vi "Unmarshal.vi"(8 "error in (no error)":errorcluster, 10 "Buffer":u8[](array[numeric]), 11 "LEN in":refnum<class "LEN.lvclass">) -> (0 "error out":errorcluster, 2 "Buffer Count":i32, 3 "LEN out":refnum<class "LEN.lvclass">)   [LabVIEW 2020, in "Protobuf RAW.lvlib" / "LEN.lvclass"]
uses:
  LEN.lvclass
  bytes/bytes.lvclass
  E:/Labview/LV 2020/Libs/LV Protobuf Raw/Source/Proto Encode/LEN Encoder/LEN.lvclass
  Message/Raw Message.lvclass
  string/string.lvclass
  E:/Labview/LV 2020/Libs/LV Protobuf Raw/Source/Proto Type Common/Proto Type Common.lvclass
  E:/Labview/LV 2020/Libs/LV Protobuf Raw/Source/Protobuf RAW/Tag/Basic Type.lvclass
  E:/Labview/LV 2020/Libs/LV Protobuf Raw/Source/Protobuf RAW/Proto Value/Proto Type.lvclass
  E:/Labview/LV 2020/Libs/LV Protobuf Raw/Source/Protobuf RAW/Type Serializer/Type Serializer.lvclass
  E:/Labview/LV 2020/Libs/LV Protobuf Raw/Source/Protobuf RAW/String Representable/String Representable.lvclass
  E:/Labview/LV 2020/Libs/LV Protobuf Raw/Source/Protobuf RAW/Wire Type Group/Wire Type Group.lvclass
  E:/Labview/LV 2020/Libs/LV Protobuf Raw/Source/Protobuf RAW/LEN Encoder/LEN.lvclass
  E:/Labview/LV 2020/Libs/LV Protobuf Raw/Source/Protobuf RAW/string/string.lvclass
  E:/Labview/LV 2020/Libs/LV Protobuf Raw/Source/Protobuf RAW/Message/Raw Message.lvclass
  E:/Labview/LV 2020/Libs/LV Protobuf Raw/Source/Protobuf RAW/bytes/bytes.lvclass
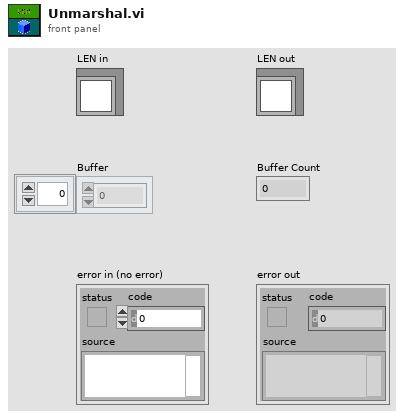
[diagram p1: front panel]
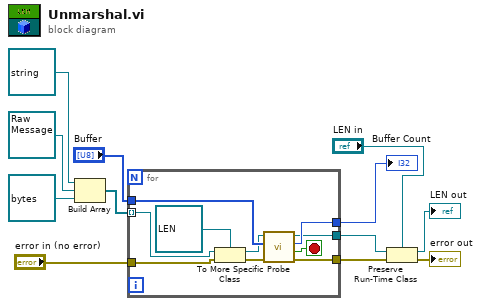
[diagram p0: block diagram]
diagram:
  n1 = Build Array(refnum<class "string.lvclass"> refnum ("Protobuf Encode.lvlib:string.lvclass"), refnum<class "Raw Message.lvclass"> refnum ("Protobuf Encode.lvlib:Raw Message.lvclass"), refnum<class "bytes.lvclass"> refnum ("Protobuf Encode.lvlib:bytes.lvclass")) -> (w1:refnum<class "Proto Type Common.lvclass">[])
  n2 = for {
    tunnel: "Buffer" -> [w21]
    tunnel: [w20] -> w10
    tunnel: w1 -> [w15] mode=indexing
    tunnel: "error in (no error)" -> [w22]
    tunnel: [w18] -> w5
    tunnel: [w17] -> w4
    stop <- w19 stop-if-true
    n3 = To More Specific Class(target class=refnum<class "LEN.lvclass"> refnum ("LEN out"), reference=w15, error in=w22) -> (specific class reference=w13:refnum<class "LEN.lvclass">, error out=w16:errorcluster)
    n4 = call-dynamic "Probe.vi"("error in (no error)"=w16, "Buffer"=w21, "LEN in"=w13) -> ("error out"=w17:errorcluster, "Valid"=w19:bool, "Buffer Count"=w20:i32, "LEN out"=w18:refnum<class "LEN.lvclass">)  [unwired: 5 in]
  }
  "Buffer Count" <- w10
  n5 = Preserve Run-Time Class(object in=w5, error in=w4, 2:"LEN in") -> (object out=→"LEN out":refnum<class "LEN.lvclass">, error out=→"error out":errorcluster)
